vi "PicoScope6000StartStreaming.vi"(0 "error in":errorcluster, 2 "handle in":i16, 3 "Enabled Channels":i16[](array[numeric]), 4 "Acquisition Settings":T1 {"Time Units" items=["Nanoseconds (ns)", "Microseconds (us)", "Milliseconds (ms)", "Seconds (s)"]; "Down-Sample Mode" items=["None", "Aggregate", "Average", "Decimate"]}) -> (6 "Channel A":i16[](array[numeric]), 7 "Channel A Min":i16[](array[numeric]), 8 "Channel B":i16[](array[numeric]), 9 "Channel B Min":i16[](array[numeric]), 10 "Channel C":i16[](array[numeric]), 11 "Channel C Min":i16[](array[numeric]), 12 "Channel D":i16[](array[numeric]), 13 "Channel D Min":i16[](array[numeric]), 14 "error out":errorcluster, 16 "handle out":i16, 17 "Sample Interval":u32)   [LabVIEW 2009]
doc: "This VI starts the oscilloscope streaming. It outputs arrays that will contain samples once PicoScope6000GetStreamingValues.vi has returned."
uses:
  ps6000.dll
  ps6000Wrap.dll
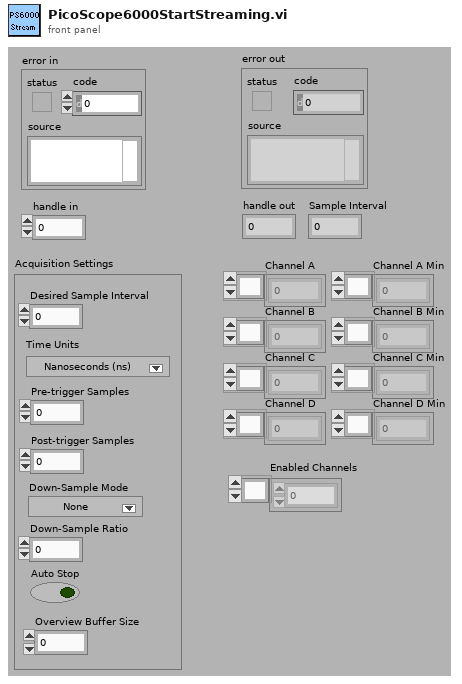
[diagram p1: front panel]
types:
  T1 = cluster{"Auto Stop":bool, "Desired Sample Interval":u32, "Pre-trigger Samples":u32, "Post-trigger Samples":u32, "Down-Sample Ratio":u32, "Down-Sample Mode":u32, "Overview Buffer Size":u32, "Time Units":u32}
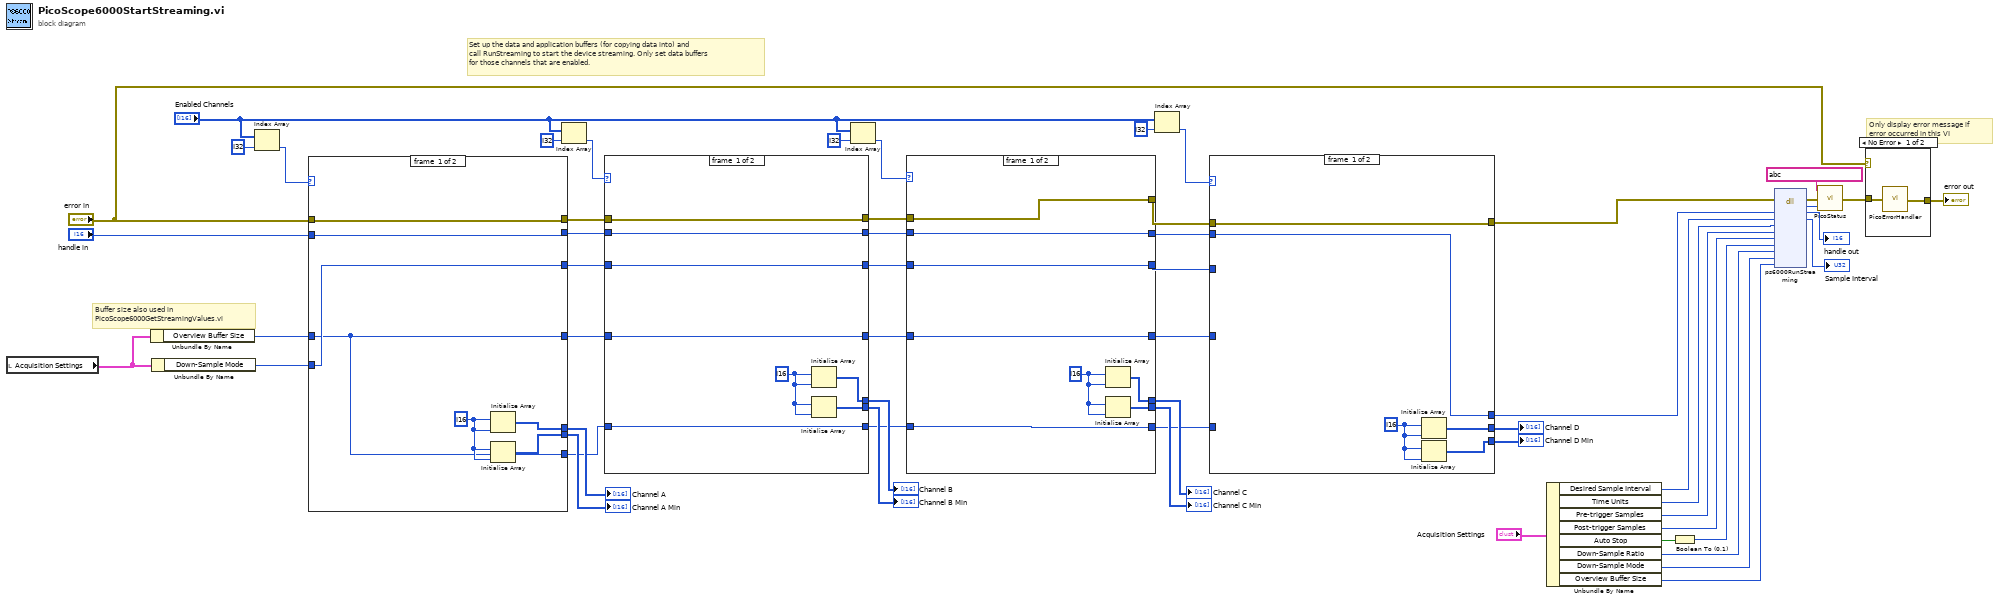
[diagram p0: block diagram]
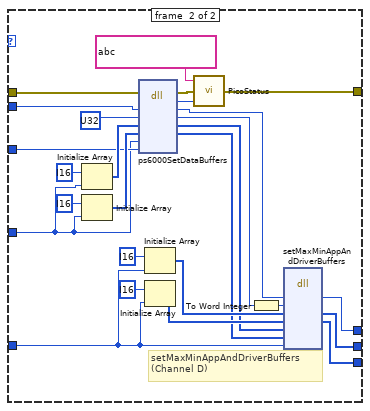
[diagram p2: hidden frame]
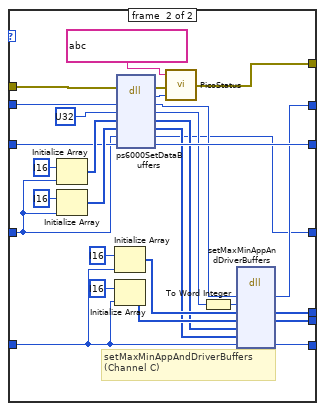
[diagram p3: hidden frame]
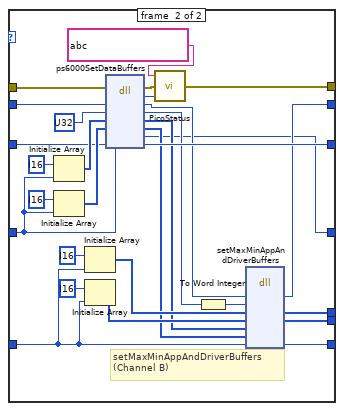
[diagram p4: hidden frame]
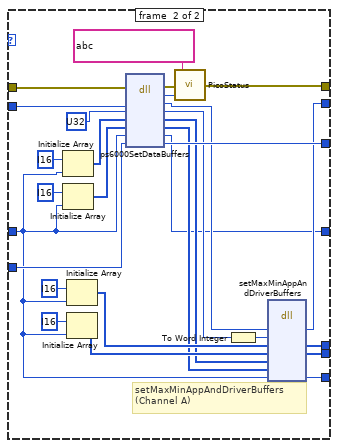
[diagram p5: hidden frame]
diagram:
  # "Only display error message if\nerror occurred in this VI"
  # "Buffer size also used in \nPicoScope6000GetStreamingValues.vi"
  # "Set up the data and application buffers (for copying data into) and \ncall RunStreaming to start the device streaming. Only set data buffers\nfor those channels that are enabled."
  n1 = local read "Acquisition Settings"() -> (w32:T1)
  n2 = Unbundle By Name(w32) -> ("Overview Buffer Size"=w14:u32)
  n3 = Unbundle By Name(w32) -> ("Down-Sample Mode"=w38:u32)
  n4 = Index Array(array="Enabled Channels", index=i32 ?) -> (element=w12:i16)
  n5 = case shown="1" w12 {
    tunnel: "handle in" -> [w62 w91]
    tunnel: [w63 w86] -> w50
    tunnel: w38 -> [w58 w81]
    tunnel: [w58 w80] -> w11
    tunnel: "error in" -> [w63 w79]
    tunnel: [w59 w74] -> w29
    tunnel: [w60 w73] -> w28
    tunnel: [w57 w72] -> w27
    tunnel: [w62 w71] -> w24
    tunnel: w14 -> [w57 w70]
    tunnel: [w57 w64] -> w10
    frame #0 {
      w61 = i16 ? ("element")
      n6 = Initialize Array(w61, w61) -> (w60:i16[])
      n7 = Initialize Array(w61, w61) -> (w59:i16[])
    }
    frame #1 {
      # "setMaxMinAppAndDriverBuffers\n(Channel A)"
      n8 = Initialize Array(i16 ? ("element"), w70) -> (w90:i16[])
      n9 = Initialize Array(i16 ? ("element"), w70) -> (w82:i16[])
      n10 = Initialize Array(i16 ? ("element"), w70) -> (w76:i16[])
      n11 = Initialize Array(i16 ? ("element"), w70) -> (w75:i16[])
      n12 = dll-call lib="PS6000.dll" fn="ps6000SetDataBuffers" ("ps3000.dll:_ps3000_open_unit@0")(error in=w79, "handle"=w91, "channel"=u32 ?, "bufferMax"=w90, "bufferMin"=w82, "bufferLth"=w70, "downSampleRatioMode"=w81) -> (error out=w87:errorcluster, "PICO_STATUS"=w88:u32, "handle"=w69:i16, "channel"=w68:u32, "bufferMax"=w66:i16[], "bufferMin"=w65:i16[], "bufferLth"=w64:u32, "downSampleRatioMode"=w80:u32)  [unwired: 2 in, 1 out]
      n13 = call "PicoStatus.vi"("PICO STATUS"=w88, "error in"=w87, "source"=string ?) -> ("error out"=w86:errorcluster)
      n14 = To Word Integer(number=w68) -> (16bit integer=w67:i16)
      n15 = dll-call lib="ps6000Wrap.dll" fn="setMaxMinAppAndDriverBuffers"("handle"=w69, "channel"=w67, "appMaxBuffer"=w76, "appMinBuffer"=w75, "driverMaxBuffer"=w66, "driverMinBuffer"=w65, "bufferLength"=w70) -> ("handle"=w71:i16, "appMaxBuffer"=w73:i16[], "appMinBuffer"=w74:i16[], "bufferLength"=w72:u32)  [unwired: 7 in, 2 out]
    }
  }
  "Channel A" <- w28
  "Channel A Min" <- w29
  n16 = Index Array(array="Enabled Channels", index=i32 ?) -> (element=w8:i16)
  n17 = case shown="1" w8 {
    tunnel: w50 -> [w99 w125]
    tunnel: [w99 w122] -> w49
    tunnel: [w97 w118] -> w37
    tunnel: w27 -> [w95 w113]
    tunnel: [w92 w112] -> w26
    tunnel: [w93 w111] -> w25
    tunnel: w24 -> [w98 w110]
    tunnel: [w98 w109] -> w23
    tunnel: [w95 w108] -> w22
    tunnel: w11 -> [w97 w102]
    tunnel: w10 -> [w96 w101]
    tunnel: [w96 w100] -> w5
    frame #0 {
      w94 = i16 ? ("element")
      n18 = Initialize Array(w94, w94) -> (w93:i16[])
      n19 = Initialize Array(w94, w94) -> (w92:i16[])
    }
    frame #1 {
      # "setMaxMinAppAndDriverBuffers\n(Channel B)"
      n20 = Initialize Array(i16 ? ("element"), w101) -> (w127:i16[])
      n21 = Initialize Array(i16 ? ("element"), w101) -> (w119:i16[])
      n22 = Initialize Array(i16 ? ("element"), w113) -> (w115:i16[])
      n23 = Initialize Array(i16 ? ("element"), w113) -> (w114:i16[])
      n24 = dll-call lib="PS6000.dll" fn="ps6000SetDataBuffers" ("ps3000.dll:_ps3000_open_unit@0")(error in=w125, "handle"=w110, "channel"=u32 ?, "bufferMax"=w127, "bufferMin"=w119, "bufferLth"=w101, "downSampleRatioMode"=w102) -> (error out=w123:errorcluster, "PICO_STATUS"=w124:u32, "handle"=w107:i16, "channel"=w106:u32, "bufferMax"=w105:i16[], "bufferMin"=w104:i16[], "bufferLth"=w100:u32, "downSampleRatioMode"=w118:u32)  [unwired: 2 in, 1 out]
      n25 = call "PicoStatus.vi"("PICO STATUS"=w124, "error in"=w123, "source"=string ?) -> ("error out"=w122:errorcluster)
      n26 = To Word Integer(number=w106) -> (16bit integer=w103:i16)
      n27 = dll-call lib="ps6000Wrap.dll" fn="setMaxMinAppAndDriverBuffers"("handle"=w107, "channel"=w103, "appMaxBuffer"=w115, "appMinBuffer"=w114, "driverMaxBuffer"=w105, "driverMinBuffer"=w104, "bufferLength"=w113) -> ("handle"=w109:i16, "appMaxBuffer"=w111:i16[], "appMinBuffer"=w112:i16[], "bufferLength"=w108:u32)  [unwired: 7 in, 2 out]
    }
  }
  "Channel B" <- w25
  "Channel B Min" <- w26
  n28 = Index Array(array="Enabled Channels", index=i32 ?) -> (element=w6:i16)
  n29 = case shown="1" w6 {
    tunnel: w49 -> [w136 w164]
    tunnel: w37 -> [w134 w160]
    tunnel: [w136 w156] -> w34
    tunnel: [w134 w154] -> w33
    tunnel: w23 -> [w135 w153]
    tunnel: w22 -> [w132 w148]
    tunnel: [w129 w147] -> w21
    tunnel: [w130 w146] -> w20
    tunnel: [w132 w145] -> w19
    tunnel: [w135 w144] -> w15
    tunnel: w5 -> [w133 w137]
    tunnel: [w133 w138] -> w4
    frame #0 {
      w131 = i16 ? ("element")
      n30 = Initialize Array(w131, w131) -> (w130:i16[])
      n31 = Initialize Array(w131, w131) -> (w129:i16[])
    }
    frame #1 {
      # "setMaxMinAppAndDriverBuffers\n(Channel C)"
      n32 = Initialize Array(i16 ? ("element"), w137) -> (w165:i16[])
      n33 = Initialize Array(i16 ? ("element"), w137) -> (w161:i16[])
      n34 = Initialize Array(i16 ? ("element"), w148) -> (w150:i16[])
      n35 = Initialize Array(i16 ? ("element"), w148) -> (w149:i16[])
      n36 = dll-call lib="PS6000.dll" fn="ps6000SetDataBuffers" ("ps3000.dll:_ps3000_open_unit@0")(error in=w164, "handle"=w153, "channel"=u32 ?, "bufferMax"=w165, "bufferMin"=w161, "bufferLth"=w137, "downSampleRatioMode"=w160) -> (error out=w157:errorcluster, "PICO_STATUS"=w158:u32, "handle"=w143:i16, "channel"=w142:u32, "bufferMax"=w140:i16[], "bufferMin"=w139:i16[], "bufferLth"=w138:u32, "downSampleRatioMode"=w154:u32)  [unwired: 2 in, 1 out]
      n37 = call "PicoStatus.vi"("PICO STATUS"=w158, "error in"=w157, "source"=string ?) -> ("error out"=w156:errorcluster)
      n38 = To Word Integer(number=w142) -> (16bit integer=w141:i16)
      n39 = dll-call lib="ps6000Wrap.dll" fn="setMaxMinAppAndDriverBuffers"("handle"=w143, "channel"=w141, "appMaxBuffer"=w150, "appMinBuffer"=w149, "driverMaxBuffer"=w140, "driverMinBuffer"=w139, "bufferLength"=w148) -> ("handle"=w144:i16, "appMaxBuffer"=w146:i16[], "appMinBuffer"=w147:i16[], "bufferLength"=w145:u32)  [unwired: 7 in, 2 out]
    }
  }
  "Channel C" <- w20
  "Channel C Min" <- w21
  n40 = Index Array(array="Enabled Channels", index=i32 ?) -> (element=w1:i16)
  n41 = case shown="1" w1 {
    tunnel: [w166 w195] -> w48
    tunnel: w34 -> [w166 w190]
    tunnel: w33 -> [_ w186]
    tunnel: w19 -> [_ w181]
    tunnel: [w167 w180] -> w18
    tunnel: [w169 w179] -> w17
    tunnel: [w168 w178] -> w16
    tunnel: w15 -> [w167 w177]
    tunnel: w4 -> [_ w171]
    frame #0 {
      w170 = i16 ? ("element")
      n42 = Initialize Array(w170, w170) -> (w169:i16[])
      n43 = Initialize Array(w170, w170) -> (w168:i16[])
    }
    frame #1 {
      # "setMaxMinAppAndDriverBuffers\n(Channel D)"
      n44 = Initialize Array(i16 ? ("element"), w171) -> (w196:i16[])
      n45 = Initialize Array(i16 ? ("element"), w171) -> (w192:i16[])
      n46 = dll-call lib="PS6000.dll" fn="ps6000SetDataBuffers" ("ps3000.dll:_ps3000_open_unit@0")(error in=w190, "handle"=w177, "channel"=u32 ?, "bufferMax"=w196, "bufferMin"=w192, "bufferLth"=w171, "downSampleRatioMode"=w186) -> (error out=w188:errorcluster, "PICO_STATUS"=w189:u32, "handle"=w176:i16, "channel"=w175:u32, "bufferMax"=w173:i16[], "bufferMin"=w172:i16[])  [unwired: 4 in, 1 out]
      n47 = Initialize Array(i16 ? ("element"), w181) -> (w183:i16[])
      n48 = Initialize Array(i16 ? ("element"), w181) -> (w182:i16[])
      n49 = call "PicoStatus.vi"("PICO STATUS"=w189, "error in"=w188, "source"=string ?) -> ("error out"=w195:errorcluster)
      n50 = To Word Integer(number=w175) -> (16bit integer=w174:i16)
      n51 = dll-call lib="ps6000Wrap.dll" fn="setMaxMinAppAndDriverBuffers"("handle"=w176, "channel"=w174, "appMaxBuffer"=w183, "appMinBuffer"=w182, "driverMaxBuffer"=w173, "driverMinBuffer"=w172, "bufferLength"=w181) -> ("handle"=w180:i16, "appMaxBuffer"=w179:i16[], "appMinBuffer"=w178:i16[])  [unwired: 8 in, 2 out]
    }
  }
  "Channel D" <- w17
  "Channel D Min" <- w16
  n52 = Unbundle By Name("Acquisition Settings") -> ("Desired Sample Interval"=w31:u32, "Time Units"=w30:u32, "Pre-trigger Samples"=w44:u32, "Post-trigger Samples"=w43:u32, "Auto Stop"=w42:bool, "Down-Sample Ratio"=w40:u32, "Down-Sample Mode"=w39:u32, "Overview Buffer Size"=w35:u32)
  n53 = Boolean To (0,1)(Boolean=w42) -> (0, 1=w45:i16)
  n54 = dll-call lib="PS6000.dll" fn="ps6000RunStreaming" ("ps3000.dll:_ps3000_open_unit@0")(error in=w48, "handle"=w18, "sampleInterval"=w31, "sampleIntervalTimeUnits"=w30, "maxPreTriggerSamples"=w44, "maxPostTriggerSamples"=w43, "autoStop"=w45, "downSampleRatio"=w40, "downSampleRatioMode"=w39, "overviewBufferSize"=w35) -> (error out=w52:errorcluster, "PICO_STATUS"=w53:u32, "handle"=→"handle out":i16, "sampleInterval"=→"Sample Interval":u32)  [unwired: 9 in, 1 out]
  n55 = call "PicoStatus.vi"("PICO STATUS"=w53, "error in"=w52, "source"=string ?) -> ("error out"=w47:errorcluster)
  n56 = case shown="No Error" "error in" {
    tunnel: [w198 w199] -> w56
    tunnel: w47 -> [w197 w199]
    frame #0 {
      n57 = call "PicoErrorHandler.vi"("error in"=w197) -> ("error out"=w198:errorcluster)
    }
    frame #1 {
    }
  }
  "error out" <- w56
